vi "GUI_passive_Visual_Test.vi"(7 "Direction":i8=45, 8 "Total trial":u16=50 min=1, 9 "Do test?":bool, 11 "lang":string) -> (1 "stop 2":bool)   [LabVIEW 2012]
uses:
  Global_var.vi
  <vilib>/Analysis/1siggen.llb/Riffle Array (I32).vi
  <vilib>/Utility/file.llb/Write To Spreadsheet File (DBL).vi
  <userlib>/dhd_sdk7/dhd_sdk7.lvlib
  <vilib>/Analysis/NI_AALBase.lvlib
panel:
  out "pos_arrray":dbl[](array[numeric])
  out "Test Type":string
  out "Trial_index":u16
  out "Correct?":bool
  out "Response":path
  out "Trajectory":path
  out "Current seq":u8
  out "Target pos":dbl[](array[numeric])
  out "flag":bool
  out "Array direction":dbl[](array[numeric])
  out "error out":errorcluster
  in  "Start?":bool
  out "Trial #":u16
  in  "stop":bool
  out "Canvas":picture
  # "degree"
  # "Is the circle moving to the right or left of the body midline?"
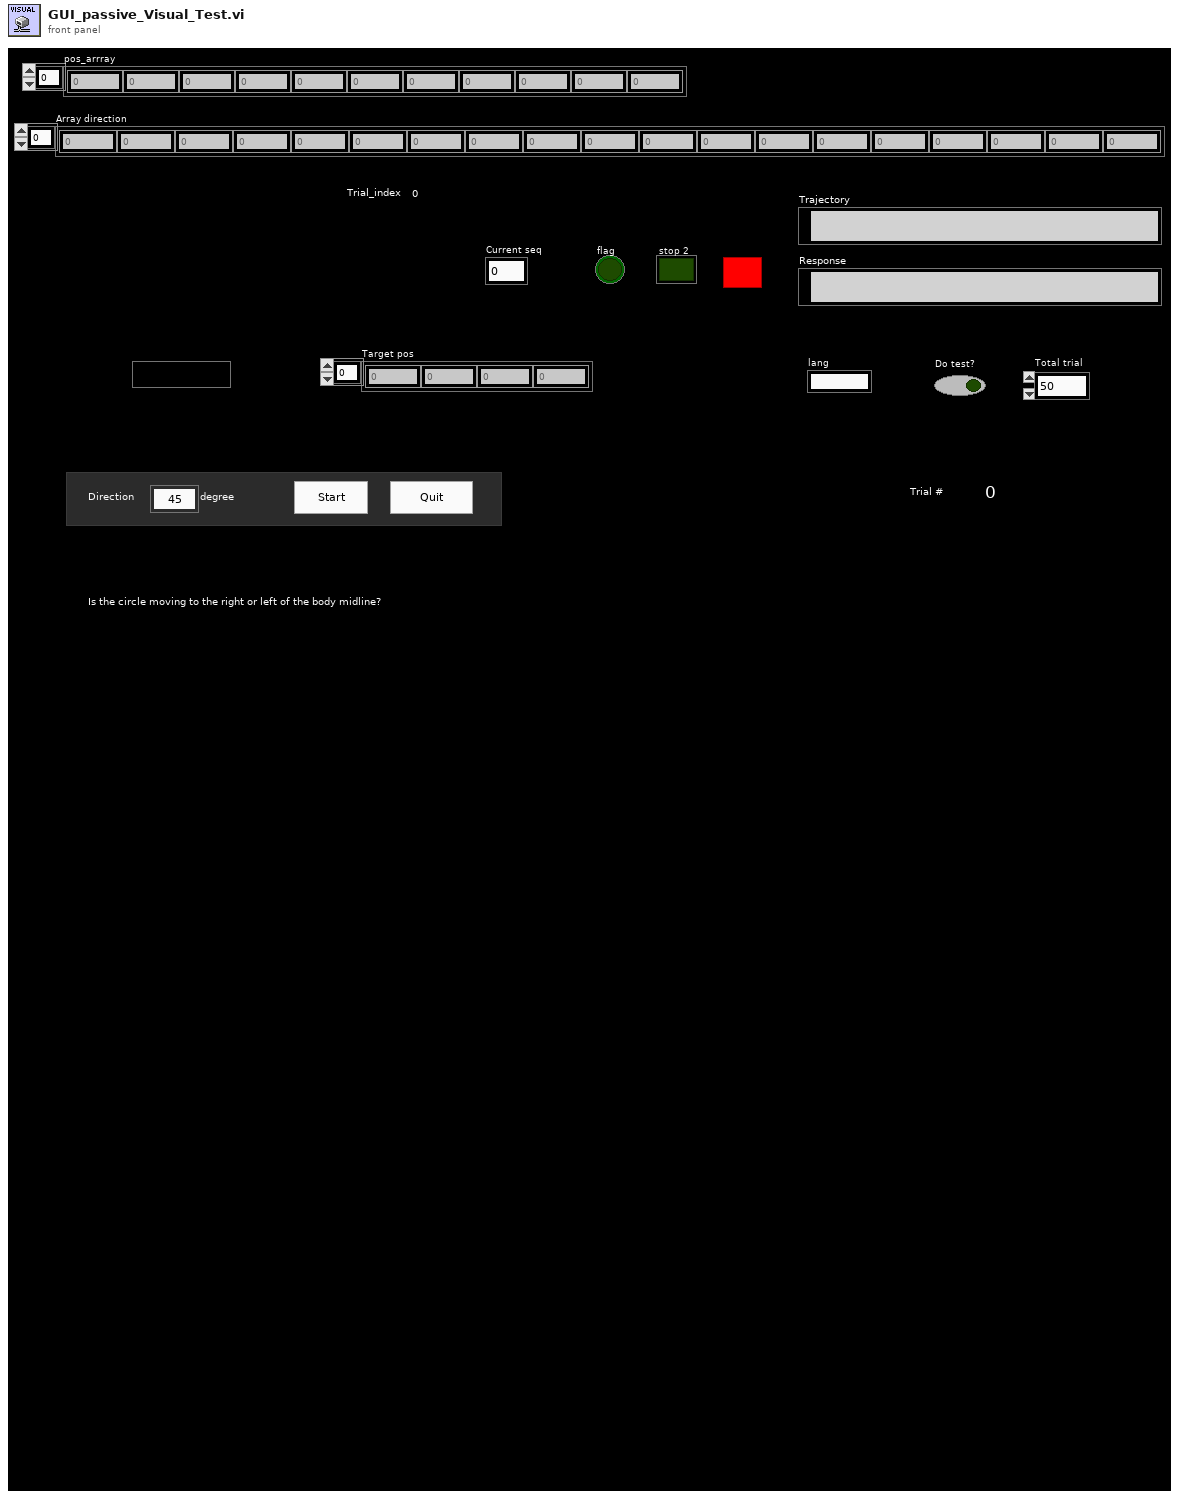
[diagram p1: front panel]
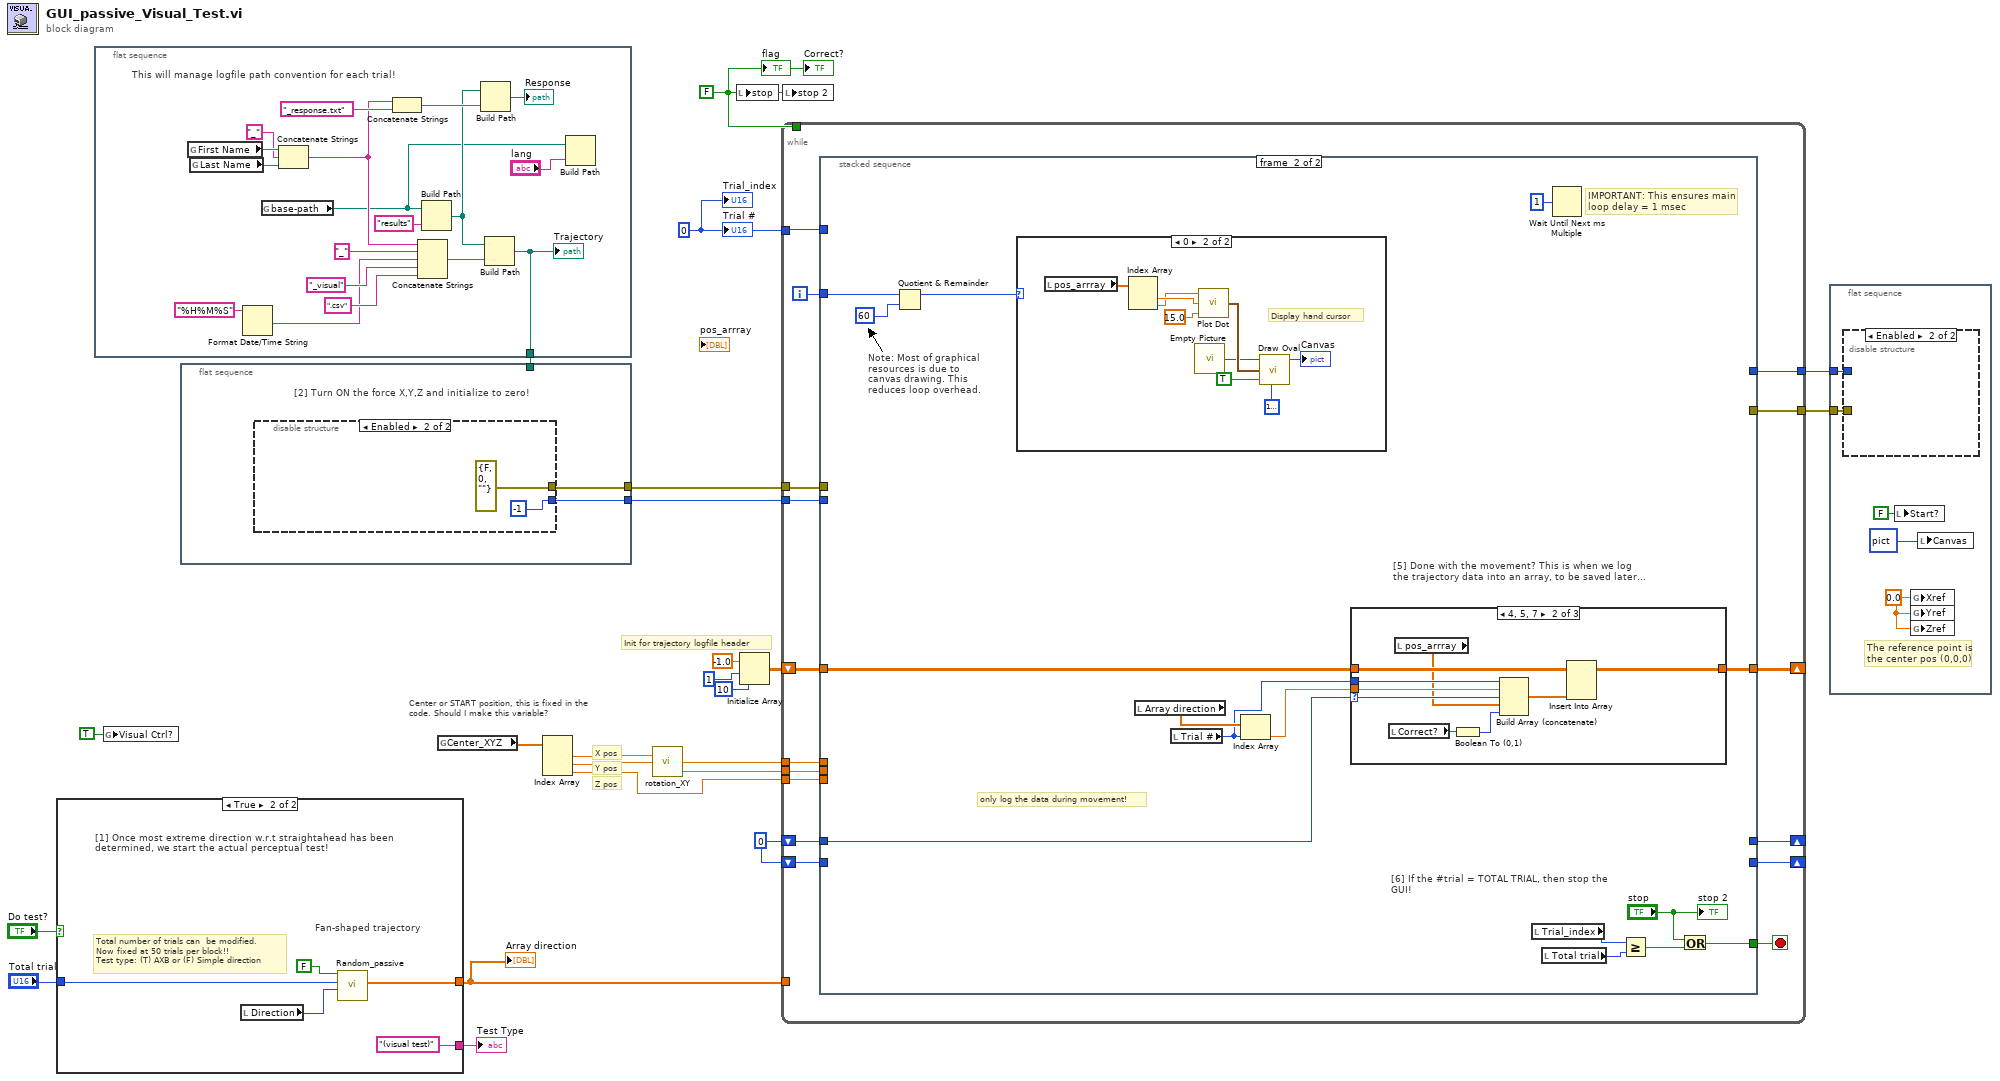
[diagram p0: block diagram]
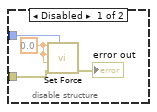
[diagram p2: hidden frame]
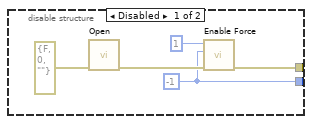
[diagram p3: hidden frame]
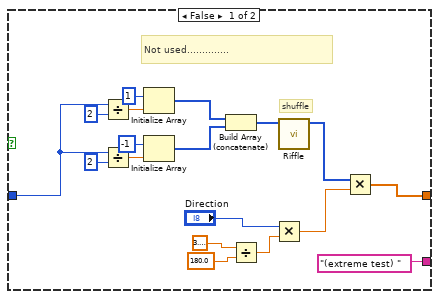
[diagram p4: hidden frame]
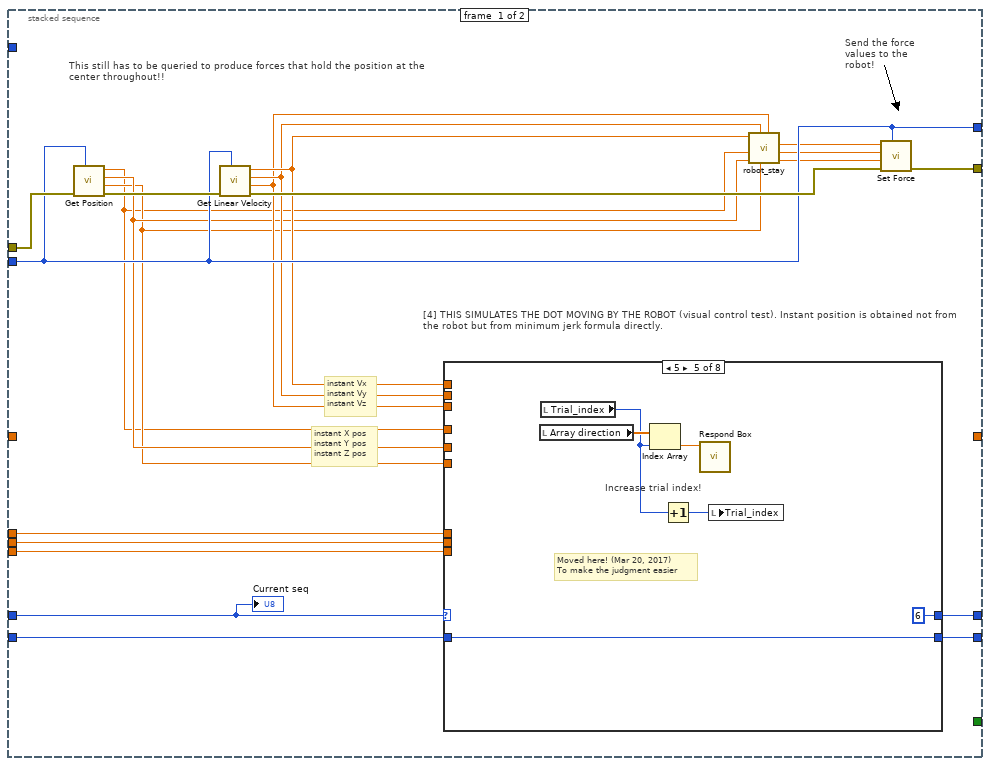
[diagram p5: hidden frame]
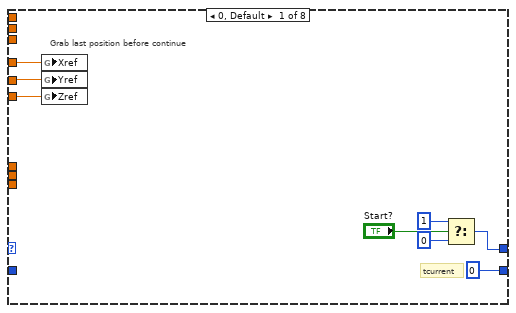
[diagram p6: hidden frame]
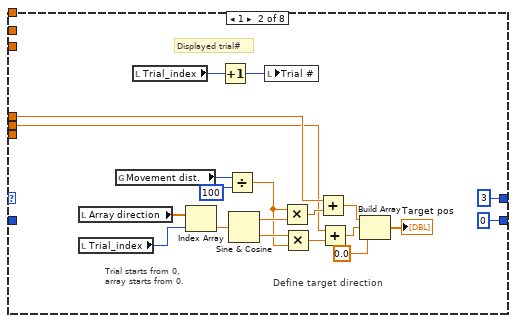
[diagram p7: hidden frame]
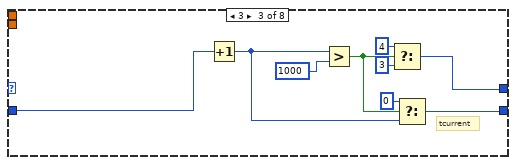
[diagram p8: hidden frame]
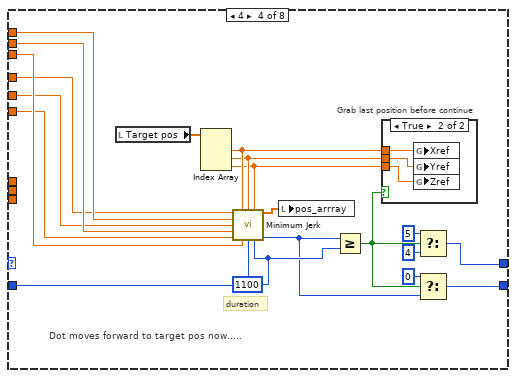
[diagram p9: hidden frame]
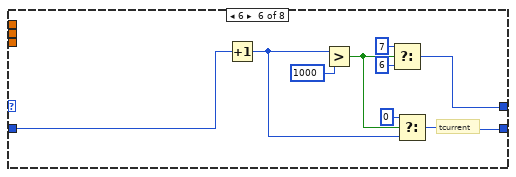
[diagram p11: hidden frame]
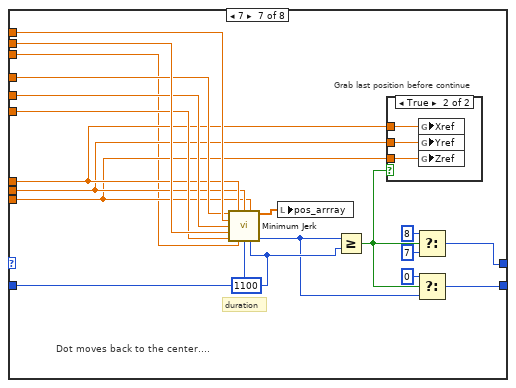
[diagram p12: hidden frame]
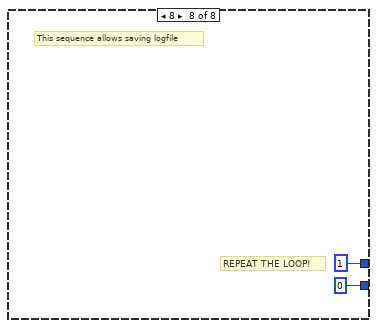
[diagram p14: hidden frame]
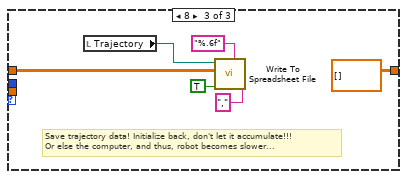
[diagram p16: hidden frame]
diagram:
  w14 = u16 0 ("y")
  w2 = FALSE ("stop")
  w23 = u16 0 ("ID")
  # "Z pos"
  # "Y pos"
  # "X pos"
  # "Center or START position, this is fixed in the code. Should I make this variable?"
  # "Init for trajectory logfile header"
  n1 = case shown="True" "Do test?" {
    tunnel: [w41 w45] -> w22
    tunnel: "Total trial" -> [w25 w44]
    tunnel: ["(extreme test) " "(visual test)"] -> w15
    frame False {
      # "Not used.............."
      # "shuffle"
      n2 = Divide(x=w25, y=u8 2) -> (x/y=w40:dbl)
      n3 = Divide(x=w25, y=u8 2) -> (x/y=w35:dbl)
      n4 = Initialize Array(i8 1 ("element"), w40) -> (w34:i8[])
      n5 = Initialize Array(i8 -1 ("element"), w35) -> (w33:i8[])
      n6 = Build Array (concatenate)(w34, w33) -> (w32:i8[])
      n7 = Divide(x=3.141592653589793, y=180.0) -> (x/y=w30:dbl)
      n8 = Multiply(x="Direction", y=w30) -> (x*y=w26:dbl)
      n9 = call-poly <vilib>:"Riffle.vi"("X"=w32) -> ("Riffled {X}"=w27:i32[])  [unwired: 8 in, 2 out]
      n10 = Multiply(x=w27, y=w26) -> (x*y=w41:dbl[])
    }
    frame True {
      # "Fan-shaped trajectory"
      # "Total number of trials can  be modified.\nNow fixed at 50 trials per block!!\nTest type: (T) AXB or (F) Simple direction"
      # "[1] Once most extreme direction w.r.t straightahead has been determined, we start the actual perceptual test!"
      n11 = local read "Direction"() -> (w46:i8)
      n12 = call "Random_passive.vi"("Degree Max."=w46, "Total trial"=w44, "Test mode\n(Simple or AXB paradigm)?"=FALSE ("Test mode\n(Simple or AXB paradigm)?")) -> ("Target"=w45:dbl[])  [unwired: 5 in, 3 out]
    }
  }
  "Array direction" <- w22
  "Test Type" <- w15
  n13 = flat-sequence {
    tunnel: [w55] -> w13
    frame #0 {
      # "This will manage logfile path convention for each trial!"
      n14 = global read "Global_var.vi" "First Name"() -> (w51:string)
      n15 = global read "Global_var.vi" "Last Name"() -> (w49:string)
      n16 = Format Date/Time String(time format string (%c)="%H%M%S") -> (date/time string=w60:string)  [unwired: 2 in]
      n17 = global read "Global_var.vi" "base-path"() -> (w47:path)
      n18 = Concatenate Strings(w51, "_" ("string"), w49) -> (w48:string)
      n19 = Concatenate Strings(w48, "_response.txt" ("string")) -> (w57:string)
      n20 = Concatenate Strings(w48, "_" ("string"), w60, "_visual" ("string"), ".csv" ("string")) -> (w64:string)
      n21 = Build Path(base path=w47, name or relative path="results") -> (appended path=w52:path)
      n22 = Build Path(base path=w52, name or relative path=w57) -> (appended path=→"Response":path)
      n23 = Build Path(base path=w52, name or relative path=w64) -> (appended path=w55:path)
      "Trajectory" <- w55
      n24 = Build Path(base path=w47, name or relative path="lang") -> ()  [unwired: 1 out]
    }
  }
  n25 = global write "Global_var.vi" "Visual Ctrl?"(TRUE ("Visual Ctrl?")) -> ()
  n26 = flat-sequence {
    tunnel: [w66] -> w11
    tunnel: [w65] -> w12
    tunnel: w13 -> [_]
    frame #0 {
      # "[2] Turn ON the force X,Y,Z and initialize to zero!"
      n27 = disable-structure shown="Enabled" {
        disable-tunnel: [w68 errorcluster {"status"=FALSE, "code"=0, "source"=""} ("error out")] -> w66
        disable-tunnel: [w67 i8 -1 ("ID")] -> w65
        frame Disabled {
          w67 = i8 -1 ("ID")
          n28 = call <userlib>:"Open.vi"("error in (no error)"=errorcluster {"status"=FALSE, "code"=0, "source"=""} ("error out")) -> ("error out"=w69:errorcluster)  [unwired: 9 in, 1 out]
          n29 = call <userlib>:"Enable Force.vi"("error in (no error)"=w69, "ID"=w67, "val"=u8 1) -> ("error out"=w68:errorcluster)  [unwired: 7 in, 1 out]
        }
        frame Enabled {
        }
      }
    }
  }
  n30 = global read "Global_var.vi" "Center_XYZ"() -> (w6:dbl[])
  n31 = Index Array(array=w6) -> (element #1=w8:dbl, element #2=w7:dbl, element #3=w3:dbl)  [unwired: 3 in]
  n32 = call "rotation_XY.vi"("x_pos"=w7, "angle"=w8) -> ("rot_y"=w4:dbl, "rot_x"=w5:dbl)  [unwired: 2 in]
  n33 = local write "stop"(w2) -> ()
  n34 = Initialize Array(-1.0 ("vz out"), 1 ("dimension size"), 10 ("dimension size")) -> (w21:dbl[][])
  n35 = while {
    shift-right: [w89] -> _
    shift-left: w23 -> [w85]
    shift-right: [w87] -> _
    shift-left: w21 -> [w86]
    tunnel: w14 -> [w83]
    shift-right: [w81] -> _
    shift-left: w23 -> [w82]
    tunnel: w2 -> [_]
    tunnel: w22 -> [_]
    tunnel: w12 -> [w80]
    tunnel: w11 -> [w79]
    tunnel: [w78] -> w10
    tunnel: [w77] -> w9
    tunnel: w5 -> [w76]
    tunnel: w4 -> [w75]
    tunnel: w3 -> [w74]
    i -> [w84]
    stop <- w88 stop-if-true
    n36 = stacked-sequence {
      tunnel: [w109 _] -> w89
      tunnel: [_ w222] -> w88
      tunnel: [_ w210] -> w87
      tunnel: w86 -> [_ w214]
      tunnel: w85 -> [w110 w211]
      tunnel: w84 -> [_ w218]
      tunnel: w83 -> [_ _]
      tunnel: w82 -> [w108 _]
      tunnel: [w107 _] -> w81
      tunnel: w80 -> [w102 _]
      tunnel: w79 -> [w104 _]
      tunnel: [w106 _] -> w78
      tunnel: [w102 _] -> w77
      tunnel: w76 -> [w101 _]
      tunnel: w75 -> [w100 _]
      tunnel: w74 -> [w99 _]
      frame #0 {
        # "instant Vx\ninstant Vy\ninstant Vz"
        # "instant X pos\ninstant Y pos\ninstant Z pos"
        # "This still has to be queried to produce forces that hold the position at the center throughout!!"
        # "Send the force values to the robot!"
        # "[4] THIS SIMULATES THE DOT MOVING BY THE ROBOT (visual control test). Instant position is obtained not from the robot but from minimum jerk formula directly."
        n37 = call <userlib>:"Get Position.vi"("ID"=w102, "error in (no error)"=w104) -> ("error out"=w105:errorcluster, "pz out"=w91:dbl, "py out"=w92:dbl, "px out"=w90:dbl)  [unwired: 5 in, 1 out]
        n38 = call <userlib>:"Get Linear Velocity.vi"("ID"=w102, "error in (no error)"=w105) -> ("error out"=w103:errorcluster, "vz out"=w93:dbl, "vy out"=w94:dbl, "vx out"=w95:dbl)  [unwired: 5 in, 1 out]
        n39 = case shown="5" w110 {
          tunnel: [w111 u8 3 ("ID") w144 w161 u8 6 ("f") w182 w188 u8 1 ("ID")] -> w109
          tunnel: w108 -> [_ _ w140 w162 w171 w178 w189 _]
          tunnel: [u16 0 ("tcurrent") u32 0 ("millisecond timer value") w142 w160 w171 w180 w187 u32 0 ("millisecond timer value")] -> w107
          tunnel: w92 -> [w117 _ _ w153 _ _ w194 _]
          tunnel: w91 -> [w116 _ _ w152 _ _ w193 _]
          tunnel: w90 -> [w115 _ _ w154 _ _ w195 _]
          tunnel: w95 -> [_ _ _ w157 _ _ w197 _]
          tunnel: w94 -> [_ _ _ w156 _ _ w196 _]
          tunnel: w93 -> [_ _ _ w155 _ _ w186 _]
          tunnel: w101 -> [_ w125 _ _ _ _ w192 _]
          tunnel: w100 -> [_ w123 _ _ _ _ w191 _]
          tunnel: w99 -> [_ _ _ _ _ _ w190 _]
          frame 0, Default {
            # "Grab last position before continue"
            # "tcurrent"
            n40 = global write "Global_var.vi" "Xref"(w115) -> ()
            n41 = global write "Global_var.vi" "Yref"(w117) -> ()
            n42 = global write "Global_var.vi" "Zref"(w116) -> ()
            n43 = Select(t=u8 1, s="Start?", f=u8 0) -> (s? t:f=w111:u8)
          }
          frame 1 {
            # "Displayed trial#"
            # "Trial starts from 0,\narray starts from 0."
            # "Define target direction"
            n44 = local read "Array direction"() -> (w134:dbl[])
            n45 = local read "Trial_index"() -> (w133:u16)
            n46 = global read "Global_var.vi" "Movement dist."() -> (w130:u8)
            n47 = local read "Trial_index"() -> (w131:u16)
            n48 = Index Array(array=w134, index=w133) -> (element=w135:dbl)
            n49 = Increment(x=w131) -> (x+1=w132:u16)
            n50 = Divide(x=w130, y=u8 100 ("x")) -> (x/y=w128:dbl)
            n51 = Sine & Cosine(0:w135) -> (1:w136:dbl, 2:w137:dbl)
            n52 = local write "Trial #"(w132) -> ()
            n53 = Multiply(x=w128, y=w136) -> (x*y=w126:dbl)
            n54 = Multiply(x=w137, y=w128) -> (x*y=w124:dbl)
            n55 = Add(x=w125, y=w126) -> (x+y=w122:dbl)
            n56 = Add(x=w123, y=w124) -> (x+y=w121:dbl)
            n57 = Build Array(w122, w121, 0.0 ("element")) -> (→"Target pos":dbl[])
          }
          frame 3 {
            # "tcurrent"
            n58 = Increment(x=w140) -> (x+1=w139:u32)
            n59 = Greater?(x=w139, y=u32 1000) -> (0:w141:bool)
            n60 = Select(t=u8 4 ("ID"), s=w141, f=u8 3) -> (s? t:f=w144:u8)
            n61 = Select(t=u8 0 ("ID"), s=w141, f=w139) -> (s? t:f=w142:u32)
          }
          frame 4 {
            w165 = u16 1100 ("duration")
            # "Grab last position before continue"
            # "duration"
            # "Dot moves forward to target pos now....."
            n62 = local read "Target pos"() -> (w151:dbl[])
            n63 = Index Array(array=w151) -> (element #1=w150:dbl, element #2=w149:dbl, element #3=w148:dbl)  [unwired: 3 in]
            n64 = call "Minimum Jerk.vi"("X"=w154, "Xfinal"=w150, "Yfinal"=w149, "Zfinal"=w148, "Vx"=w157, "Y"=w153, "Vy"=w156, "Z"=w152, "Vz"=w155, "current_n"=w162, "duration"=w165) -> ("Pos_dest"=w159:dbl[], "n out"=w163:u16)  [unwired: 3 out]
            n65 = local write "pos_arrray"(w159) -> ()
            n66 = Greater Or Equal?(x=w163, y=w165) -> (x >= y?=w158:bool)
            n67 = case shown="True" w158 {
              tunnel: w150 -> [_ w170]
              tunnel: w149 -> [_ w169]
              tunnel: w148 -> [_ w168]
              frame False {
              }
              frame True {
                n68 = global write "Global_var.vi" "Xref"(w170) -> ()
                n69 = global write "Global_var.vi" "Yref"(w169) -> ()
                n70 = global write "Global_var.vi" "Zref"(w168) -> ()
              }
            }
            n71 = Select(t=u8 5 ("ID"), s=w158, f=u8 4) -> (s? t:f=w161:u8)
            n72 = Select(t=u8 0 ("ID"), s=w158, f=w163) -> (s? t:f=w160:u16)
          }
          frame 5 {
            # "Moved here! (Mar 20, 2017)\nTo make the judgment easier"
            # "Increase trial index!"
            n73 = local read "Array direction"() -> (w176:dbl[])
            n74 = local read "Trial_index"() -> (w173:u16)
            n75 = Index Array(array=w176, index=w173) -> (element=w175:dbl)
            n76 = Increment(x=w173) -> (x+1=w174:u16)
            n77 = call "Respond Box.vi"("target"=w175) -> ()  [unwired: 5 in, 3 out]
            n78 = local write "Trial_index"(w174) -> ()
          }
          frame 6 {
            # "tcurrent"
            n79 = Increment(x=w178) -> (x+1=w177:u32)
            n80 = Greater?(x=w177, y=u32 1000) -> (0:w179:bool)
            n81 = Select(t=u8 7 ("ID"), s=w179, f=u8 6) -> (s? t:f=w182:u8)
            n82 = Select(t=u8 0 ("ID"), s=w179, f=w177) -> (s? t:f=w180:u32)
          }
          frame 7 {
            w202 = u16 1100 ("duration")
            # "Grab last position before continue"
            # "duration"
            # "Dot moves back to the center...."
            n83 = call "Minimum Jerk.vi"("X"=w195, "Xfinal"=w192, "Yfinal"=w191, "Zfinal"=w190, "Vx"=w197, "Y"=w194, "Vy"=w196, "Z"=w193, "Vz"=w186, "current_n"=w189, "duration"=w202) -> ("Pos_dest"=w199:dbl[], "n out"=w200:u16)  [unwired: 3 out]
            n84 = local write "pos_arrray"(w199) -> ()
            n85 = Greater Or Equal?(x=w200, y=w202) -> (x >= y?=w198:bool)
            n86 = case shown="True" w198 {
              tunnel: w192 -> [_ w207]
              tunnel: w191 -> [_ w206]
              tunnel: w190 -> [_ w205]
              frame False {
              }
              frame True {
                n87 = global write "Global_var.vi" "Xref"(w207) -> ()
                n88 = global write "Global_var.vi" "Yref"(w206) -> ()
                n89 = global write "Global_var.vi" "Zref"(w205) -> ()
              }
            }
            n90 = Select(t=u8 8 ("ID"), s=w198, f=u8 7) -> (s? t:f=w188:u8)
            n91 = Select(t=u8 0 ("ID"), s=w198, f=w200) -> (s? t:f=w187:u16)
          }
          frame 8 {
            # "This sequence allows saving logfile"
            # "REPEAT THE LOOP!"
          }
        }
        n92 = call "robot_stay.vi"("Vz"=w93, "Z"=w91, "Vy"=w94, "Y"=w92, "X"=w90, "Vx"=w95) -> ("Fz"=w96:dbl, "Fy"=w97:dbl, "Fx"=w98:dbl)  [unwired: 3 in]
        n93 = call <userlib>:"Set Force.vi"("ID"=w102, "error in (no error)"=w103, "fz"=w96, "fy"=w97, "fx"=w98) -> ("error out"=w106:errorcluster)  [unwired: 5 in, 1 out]
        "Current seq" <- w110
      }
      frame #1 {
        # "Note: Most of graphical resources is due to canvas drawing. This\nreduces loop overhead."
        # "IMPORTANT: This ensures main \nloop delay = 1 msec"
        # "only log the data during movement!"
        # "[5] Done with the movement? This is when we log\nthe trajectory data into an array, to be saved later..."
        # "[6] If the #trial = TOTAL TRIAL, then stop the GUI!"
        n94 = Quotient & Remainder(x=w218, y=60) -> (x-y*floor(x/y)=w220:i32)  [unwired: 1 out]
        n95 = case shown="0" w220 {
          frame 1, Default {
            # "Nothng would be displayed here..."
          }
          frame 0 {
            # "Display hand cursor"
            n96 = local read "pos_arrray"() -> (w244:dbl[])
            n97 = Index Array(array=w244) -> (element #1=w243:dbl, element #2=w242:dbl)  [unwired: 2 in]
            n98 = call "Empty Picture"() -> ("empty picture"=w241:picture)
            n99 = call "Plot Dot.vi"("Diameter"=15.0 ("Size"), "Y"=w243, "X"=w242) -> ("Cluster"=w245:cluster{dbl, dbl, dbl, dbl})
            n100 = call <vilib>:"Draw Oval.vi"("picture"=w241, "rect"=w245, "fill?(F)"=TRUE, "color(black)"=u32 16777226) -> ("new picture"=→"Canvas":picture)  [unwired: 5 in]
          }
        }
        n101 = local read "Array direction"() -> (w217:dbl[])
        n102 = local read "Trial #"() -> (w213:u16)
        n103 = Index Array(array=w217, index=w213) -> (element=w212:dbl)
        n104 = case shown="4, 5, 7" w211 {
          selector: w211 -> [_ w229 _]
          tunnel: [w225 w233 dbl[][] []] -> w210
          tunnel: w214 -> [w225 w232 w237]
          tunnel: w212 -> [_ w231 _]
          tunnel: w213 -> [_ w230 _]
          frame 0, Default {
          }
          frame 4, 5, 7 {
            n105 = local read "Correct?"() -> (w228:bool)
            n106 = local read "pos_arrray"() -> (w226:dbl[])
            n107 = Boolean To (0,1)(Boolean=w228) -> (0, 1=w227:i16)
            n108 = Build Array (concatenate)(w230, w231, w229, w226, w227) -> (w234:dbl[])
            n109 = Insert Into Array(array=w232, new element=w234) -> (w233:dbl[][])  [unwired: 2 in]
          }
          frame 8 {
            # "Save trajectory data! Initialize back, don't let it accumulate!!!\nOr else the computer, and thus, robot becomes slower..."
            n110 = local read "Trajectory"() -> (w240:path)
            n111 = call-poly <vilib>:"Write To Spreadsheet File.vi"("delimiter (\\t)"="," ("delimiter (\\t)"), "format (%.3f)"="%.6f", "append to file? (new file:F)"=TRUE, "2D data"=w237, "file path (dialog if empty)"=w240) -> ()  [unwired: 3 in, 1 out]
          }
        }
        n112 = local read "Trial_index"() -> (w223:u16)
        n113 = local read "Total trial"() -> (w216:u16)
        n114 = Wait Until Next ms Multiple(millisecond multiple=u32 1) -> ()  [unwired: 1 out]
        n115 = Greater Or Equal?(x=w223, y=w216) -> (x >= y?=w224:bool)
        n116 = Or(x="stop", y=w224) -> (x .or. y?=w222:bool)
        "stop 2" <- "stop"
      }
    }
  }
  n117 = local write "stop 2"(w2) -> ()
  n118 = flat-sequence {
    tunnel: w10 -> [w254]
    tunnel: w9 -> [w253]
    frame #0 {
      w250 = 0.0 ("Xref")
      # "The reference point is\nthe center pos (0,0,0)"
      n119 = disable-structure shown="Enabled" {
        disable-tunnel: w254 -> [w258 _]
        disable-tunnel: w253 -> [w257 _]
        frame Disabled {
          w255 = 0.0 ("fx")
          n120 = call <userlib>:"Set Force.vi"("ID"=w257, "error in (no error)"=w258, "fz"=w255, "fy"=w255, "fx"=w255) -> ("error out"=→"error out":errorcluster)  [unwired: 5 in, 1 out]
        }
        frame Enabled {
        }
      }
      n121 = local write "Start?"(FALSE ("start")) -> ()
      n122 = global write "Global_var.vi" "Xref"(w250) -> ()
      n123 = global write "Global_var.vi" "Yref"(w250) -> ()
      n124 = global write "Global_var.vi" "Zref"(w250) -> ()
      n125 = local write "Canvas"(picture data[5B] ("Canvas")) -> ()
    }
  }
  "flag" <- w2
  "Trial #" <- w14
  "Correct?" <- w2
  "Trial_index" <- w14
